vi "DefineFont.vi"(8 "error in (no error)":errorcluster, 10 "Font Cluster":T1={"familyName"="Arial", "emSize"=0.3, "style"=enum."Regular"}) -> (0 "error out":errorcluster, 3 "Font out":refnum<class "Font.lvclass">)   [LabVIEW 2016, in "DataGrid.lvlib" / "Font.lvclass"]
uses:
  <userlib>/LabVIEWdotNetDataGrid/source/Font/Font.lvclass
  <userlib>/LabVIEWdotNetDataGrid/source/Font/Font Cluster.ctl
  System.Drawing
  <userlib>/LabVIEWdotNetDataGrid/source/Font/Font.lvclass/Font.ctl
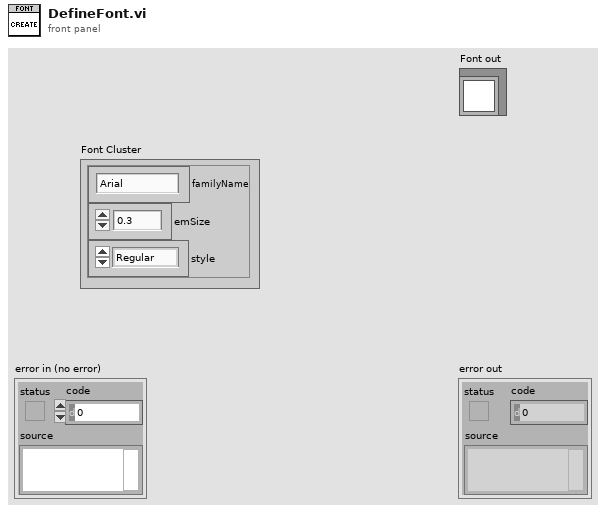
[diagram p1: front panel]
types:
  T1 = typedef "DataGrid.lvlib/Font.lvclass/Font Cluster.ctl" = cluster{"familyName":string, "emSize":sgl, "style":enum16{"Regular", "Bold", "Italic", "Underline", "Strikeout"}}
  T2 = enum16{"Regular", "Bold", "Italic", "Underline", "Strikeout"}
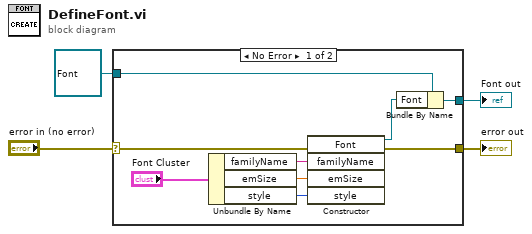
[diagram p0: block diagram]
diagram:
  n1 = case shown="No Error" "error in (no error)" {
    selector: "error in (no error)" -> [w12 w15]
    tunnel: [w9 w15] -> w3
    tunnel: [w10 w14] -> w1
    tunnel: refnum<class "Font.lvclass"> refnum ("Font in") -> [w11 w14]
    frame No Error {
      n2 = Unbundle By Name("Font Cluster") -> ("familyName"=w7:string, "emSize"=w6:sgl, "style"=w5:T2)
      n3 = constructor class="Font"(error in=w12, "familyName"=w7, "emSize"=w6, "style"=w5) -> (reference out=w13:refnum<k24>, error out=w9:errorcluster)  [unwired: 2 in, 4 out]
      n4 = Bundle By Name(cluster=w11, "Font"=w13) -> (w10:refnum<class "Font.lvclass">)
    }
    frame Error {
    }
  }
  "error out" <- w3
  "Font out" <- w1
